vi "Read Resource.vi"(8 "error in (no error)":errorcluster, 11 "PowerSupplyVisa-Fix in":refnum<class "PowerSupplyVisa-Fix.lvclass">) -> (0 "error out":errorcluster, 2 "Resource":refnum<visa-resource-name>, 3 "PowerSupplyVisa-Fix out":refnum<class "PowerSupplyVisa-Fix.lvclass">)   [LabVIEW 2020, in "LAF2024Q2.lvlib" / "PowerSupplyVisa-Fix.lvclass"]
uses:
  PowerSupplyVisa-Fix.lvclass
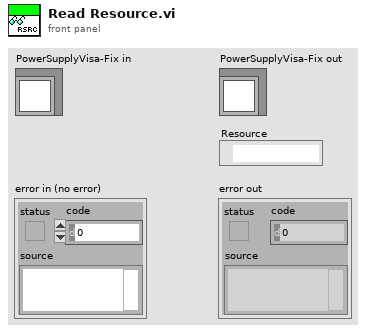
[diagram p1: front panel]
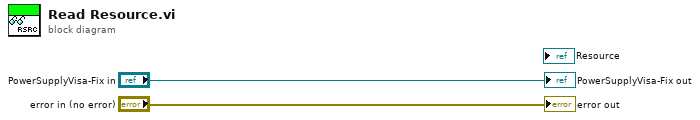
[diagram p0: block diagram]
diagram:
  "error out" <- "error in (no error)"
  "PowerSupplyVisa-Fix out" <- "PowerSupplyVisa-Fix in"
